vi "PXI-General Init and Create Tasks.vi"(0 "AO Channels":i32[](array[numeric]), 7 "AI Channels":i32[](array[numeric]), 11 "error in (no error)":errorcluster) -> (4 "Task Specification Array":T1[](array[typedef]), 15 "error out":errorcluster)   [LabVIEW 2015]
uses:
  Type Defs/Task Struct (compact).ctl
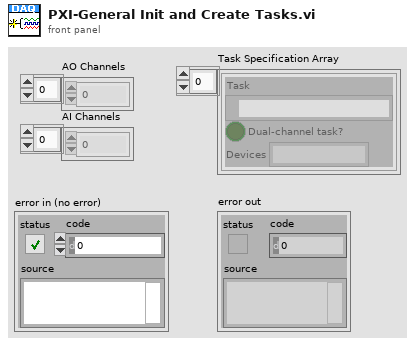
[diagram p1: front panel]
types:
  T1 = typedef "Task Struct (compact).ctl" = cluster{"Task":refnum<k21>, "Dual-channel task?":bool, "Devices":string}
  T2 = cluster{"DAQChan to PhysDev":i32[][], "PhysDev to DAQChan":i32[][]}
  T3 = typedef "Channel Struct.ctl" = cluster{"Channel name":string, "Vmax":dbl, "Vmin":dbl, "Rate":dbl, "Terminal configuration":i32, "Physical Channel":tag, "Regenerate":bool}
  T4 = typedef "Task Specification Struct.ctl" = cluster{"Task name":string, "Task":refnum<k21>, "Dual-channel task?":bool, "Channels":T3[]}
  T5 = cluster{"Task":refnum<k21>, "Dual-channel task?":bool, string}
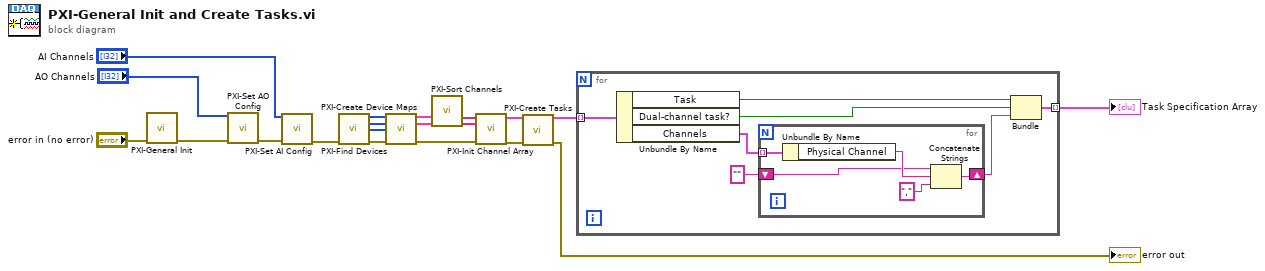
[diagram p0: block diagram]
diagram:
  n1 = call "PXI-General Init.vi"("error in (no error)"="error in (no error)") -> ("error out"=w7:errorcluster)  [unwired: 10 in]
  n2 = call "PXI-Set AO Config.vi"("AO Channels"="AO Channels", "error in (no error)"=w7) -> ("error out"=w5:errorcluster)  [unwired: 13 in]
  n3 = call "PXI-Set AI Config.vi"("AI Channels"="AI Channels", "error in (no error)"=w5) -> ("error out"=w3:errorcluster)  [unwired: 13 in]
  n4 = call "PXI-Find Devices.vi"("error in (no error)"=w3) -> ("Num AO"=w12:i32[], "Num AI"=w13:i32[], "Slot Num"=w10:u32[], "error out"=w11:errorcluster)  [unwired: 11 in]
  n5 = call "PXI-Create Device Maps.vi"("Num AO"=w12, "Num AI"=w13, "Slot Num"=w10, "error in (no error)"=w11) -> ("AO Map"=w14:T2, "AI Map"=w15:T2, "error out"=w20:errorcluster)  [unwired: 9 in]
  n6 = call "PXI-Sort Channels.vi"("AO Map"=w14, "AI Map"=w15) -> ("Sorted channel names"=w16:string[], "Sorted physical channels"=w17:tag[])  [unwired: 12 in]
  n7 = call "PXI-Init Channel Array.vi"("Sorted channel names"=w16, "Sorted physical channels"=w17, "error in (no error)"=w20) -> ("Channel Array"=w19:T3[], "error out"=w18:errorcluster)  [unwired: 11 in]
  n8 = call "PXI-Create Tasks.vi"("I/O Channels"=w19, "error in (no error)"=w18) -> ("Task Specification Array"=w2:T4[], "error out"=→"error out":errorcluster)  [unwired: 12 in]
  n9 = for {
    tunnel: w2 -> [w27] mode=indexing
    tunnel: [w24] -> w1 mode=indexing
    n10 = Unbundle By Name(w27) -> ("Task"=w25:refnum<k21>, "Dual-channel task?"=w26:bool, "Channels"=w23:T3[])
    n11 = for {
      tunnel: w23 -> [w32] mode=indexing
      shift-right: [w31] -> w21
      shift-left: "" -> [w29]
      n12 = Unbundle By Name(w32) -> ("Physical Channel"=w30:tag)
      n13 = Concatenate Strings(w29, w30, ",") -> (w31:string)
    }
    n14 = Bundle("Task"=w25, "Dual-channel task?"=w26, w21) -> (w24:T5)  [unwired: 1 in]
  }
  "Task Specification Array" <- w1
